vi "Send TIME Command.vi"(8 "error in (no error)":errorcluster, 11 "Time Stamp":timestamp) -> (0 "error out":errorcluster)   [LabVIEW 2014]
doc: "Sends TIME command to myRIO. This tells the myRIO to reset its clock according to the Time Stamp input."
uses:
  Controls/UDP Reference Action Enum.ctl
panel:
  out "concatenated string":string
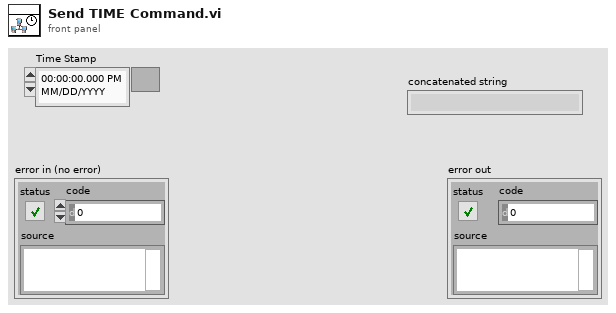
[diagram p1: front panel]
types:
  T1 = typedef "UDP Reference Action Enum.ctl" = enum16{"Set", "Get"}
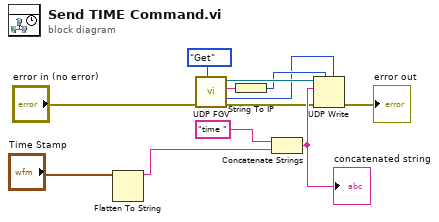
[diagram p0: block diagram]
diagram:
  n1 = Flatten To String(anything="Time Stamp") -> (data string=w1:string)  [unwired: 3 in, 2 out]
  n2 = call "UDP FGV.vi"("Action"=UDP_Reference_Action_Enum."Get", "error in (no error)"="error in (no error)") -> ("error out"=w8:errorcluster, "Port Out"=w3:u16, "IP Address out"=w5:string, "connection ID out"=w9:refnum<k16>)  [unwired: 6 in]
  n3 = String To IP(1:w5) -> (0:w4:u32)
  n4 = Concatenate Strings("time ", w1) -> (w12:string)
  "concatenated string" <- w12
  n5 = UDP Write(address=w4, port or service name=w3, connection ID=w9, data in=w12, 8:w8) -> (error out=→"error out":errorcluster)  [unwired: 1 in, 1 out]
